vi "set_visitor.vi"(0 "HGF_FGV_Visitor":refnum<class "HGF_FGV_Visitor.lvclass">, 2 "visitor":refnum<class "HGF_Visitor.lvclass">, 5 "error in (no error)":errorcluster) -> (14 "dup HGF_FGV_Visitor":refnum<class "HGF_FGV_Visitor.lvclass">, 19 "error out":errorcluster)   [LabVIEW 2012, in "HGF_FGV.lvlib" / "HGF_FGV_Visitor.lvclass"]
doc: "Set HGF_Visitor."
uses:
  HGF_FGV_Visitor.lvclass
  HGF_Visitor/HGF_Visitor.lvclass
  HGF_FGV_Visitor.lvclass/HGF_FGV_Visitor.ctl
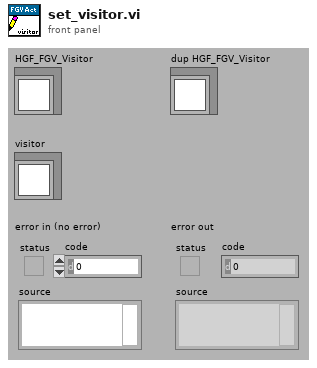
[diagram p1: front panel]
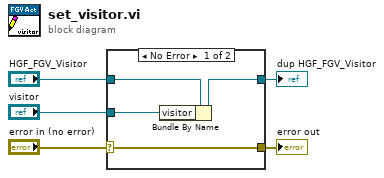
[diagram p0: block diagram]
diagram:
  n1 = case shown="No Error" "error in (no error)" {
    selector: "error in (no error)" -> [w9 w10]
    tunnel: [w9 w10] -> w4
    tunnel: [w7 w11] -> w2
    tunnel: "HGF_FGV_Visitor" -> [w8 w11]
    tunnel: "visitor" -> [w6 _]
    frame No Error {
      n2 = Bundle By Name(cluster=w8, "visitor"=w6) -> (w7:refnum<class "HGF_FGV_Visitor.lvclass">)
    }
    frame Error {
    }
  }
  "error out" <- w4
  "dup HGF_FGV_Visitor" <- w2
